vi "轴心轨迹.vi"() -> ()   [LabVIEW 2010]
uses:
  Instance           1 16Saved   轴心轨迹 .vi
  Instance           3 16Saved   轴心轨迹 .vi
  Instance           2 16Saved   轴心轨迹 .vi
panel:
  out "X振动波形":dbl[](graph)
  out "Y振动波形":dbl[](graph)
  out "轴心轨迹(μm)":cluster{dbl[], dbl[]}(graph)
  in  "stop (F)":bool
  # "轴心轨迹测量实验"
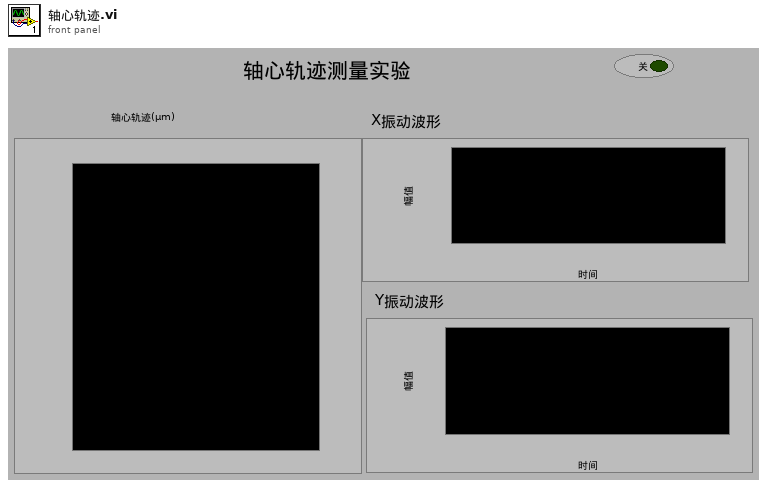
[diagram p1: front panel]
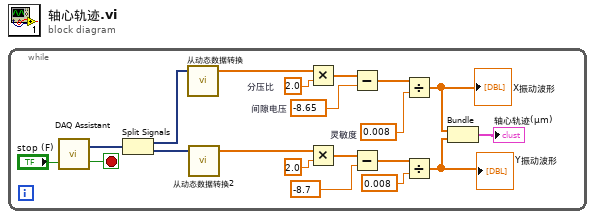
[diagram p0: block diagram]
diagram:
  n1 = while {
    stop <- w19 stop-if-true
    w9 = -8.65  # 间隙电压
    w14 = 2.0  # 分压比
    w17 = 0.008  # 灵敏度
    n2 = call "DAQ Assistant"("stop (F)"="stop (F)") -> ("data"=w18:dynamicdata, "stopped"=w19:bool)  [unwired: 15 in, 2 out]
    n3 = Split Signals(w18) -> (w7:dynamicdata, w6:dynamicdata)  [unwired: 2 in]
    n4 = call "从动态数据转换"("Dynamic Data Type"=w7) -> ("Array"=w3:dbl[])  [unwired: 3 in]
    n5 = call "从动态数据转换2"("Dynamic Data Type"=w6) -> ("Array"=w4:dbl[])  [unwired: 3 in]
    n6 = Multiply(x=w3, y=w14) -> (x*y=w15:dbl[])
    n7 = Multiply(x=w4, y=2.0) -> (x*y=w12:dbl[])
    n8 = Subtract(x=w15, y=w9) -> (x-y=w16:dbl[])
    n9 = Subtract(x=w12, y=-8.7 ("间隙电压 2")) -> (x-y=w11:dbl[])
    n10 = Divide(x=w16, y=w17) -> (x/y=w2:dbl[])
    "X振动波形" <- w2
    n11 = Divide(x=w11, y=0.008) -> (x/y=w1:dbl[])
    "Y振动波形" <- w1
    n12 = Bundle(w2, w1) -> (→"轴心轨迹(μm)":cluster{dbl[], dbl[]})  [unwired: 1 in]
  }
